vi "__VI to Create Object DVR.vi"() -> ()   [LabVIEW 2016, in "SLL Class DVR API Generator.lvlib"]
uses:
  SLL Class DVR API Generator.lvlib
  Example/My Sample Class.lvclass
panel:
  in  "My Sample Class.lvclass":refnum<class "My Sample Class.lvclass">
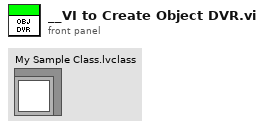
[diagram p1: front panel]
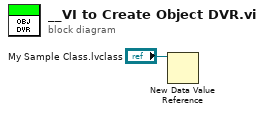
[diagram p0: block diagram]
diagram:
  n1 = New Data Value Reference(data value="My Sample Class.lvclass") -> ()  [unwired: 1 in, 2 out]
